vi "HEWH WT210 Data Save.vi"(10 "MW100 Data":string[][](array[string]), 11 "output cluster":T1={"Current (A):Element 1"=236.2, "Current (A):Element 2"=17.749, "Power (W):Sigma"=4192.0, "Watt Hours (Wh):Sigma"=0.0, "Voltage (V):Element 2"=236.2, "Voltage (V):Element 1"=236.2, "Current Crest Factor:Element 1"=0.0, "Current Crest Factor:Element 2"=0.0, "Voltage Harmonic (%):Element 1"=0.0, "Voltage Harmonic (%):Element 2"=0.0, "Voltage Crest Factor:Element 1"=0.0, "Voltage Crest Factor:Element 2"=0.0, "Time:Element 1"=0.0, "Frequency (Hz):Element 1"=0.0, "Apparent Power (VA):Element 1"=0.0, "Apparent Power (VA):Element 2"=0.0, "Power Factor:Element 1"=0.0, "Power Factor:Element 2"=0.0, "Max Watt Hours"=0.0, "Voltage (V):Element 2 Avg"=0.0, "Voltage (V):Element 1 Avg"=0.0} {"Voltage (V):Element 1 Avg" format="%.3g"; "Voltage (V):Element 2 Avg" format="%.3g"; "Max Watt Hours" format="%.3g"; "Power Factor:Element 2" format="%.3g"; "Power Factor:Element 1" format="%.3g"; "Apparent Power (VA):Element 2" format="%.3g"; "Apparent Power (VA):Element 1" format="%.3g"; "Frequency (Hz):Element 1" format="%.3g"; "Time:Element 1" format="%.3g"; "Voltage Crest Factor:Element 2" format="%.3g"; "Voltage Crest Factor:Element 1" format="%.3g"; "Voltage Harmonic (%):Element 2" format="%.3g"; "Voltage Harmonic (%):Element 1" format="%.3g"; "Current Crest Factor:Element 2" format="%.3g"; "Current Crest Factor:Element 1" format="%.3g"; "Voltage (V):Element 1" format="%.3g"; "Voltage (V):Element 2" format="%.3g"; "Watt Hours (Wh):Sigma" format="%.3f"; "Power (W):Sigma" format="%.3g"; "Current (A):Element 2" format="%.3e"; "Current (A):Element 1" format="%.3e"}) -> (3 "MW100 Data":string[][](array[string]))   [LabVIEW 2019]
uses:
  Utility/Type Definitions/UTILITY Power Data.ctl
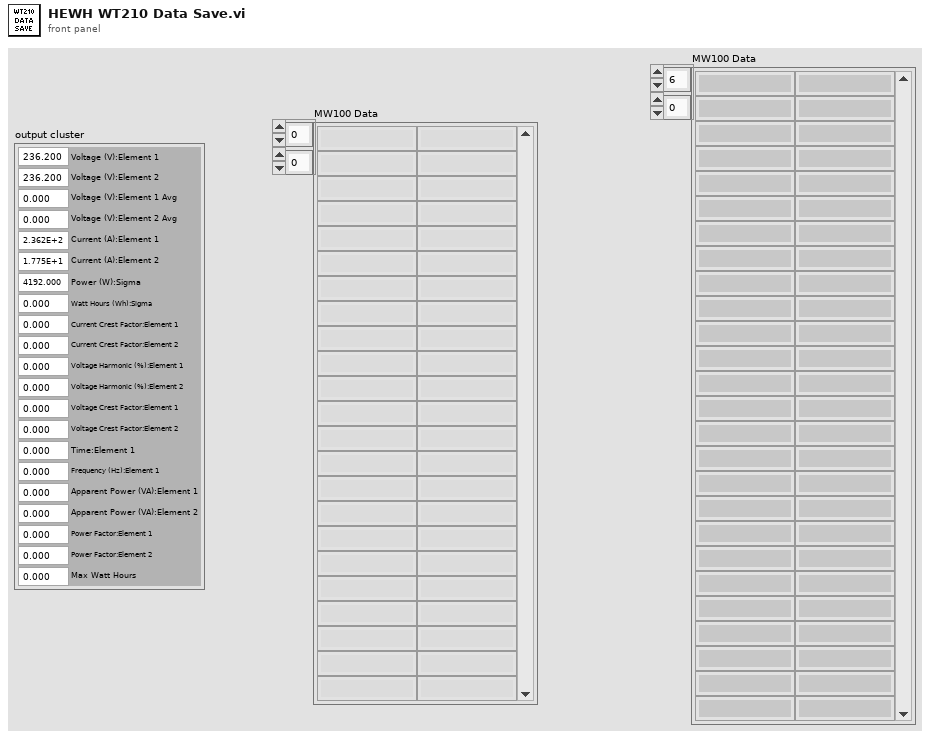
[diagram p1: front panel]
types:
  T1 = typedef "UTILITY Power Data.ctl" = cluster{"Current (A):Element 1":dbl, "Current (A):Element 2":dbl, "Power (W):Sigma":dbl, "Watt Hours (Wh):Sigma":dbl, "Voltage (V):Element 2":dbl, "Voltage (V):Element 1":dbl, "Current Crest Factor:Element 1":dbl, "Current Crest Factor:Element 2":dbl, "Voltage Harmonic (%):Element 1":dbl, "Voltage Harmonic (%):Element 2":dbl, "Voltage Crest Factor:Element 1":dbl, "Voltage Crest Factor:Element 2":dbl, "Time:Element 1":dbl, "Frequency (Hz):Element 1":dbl, "Apparent Power (VA):Element 1":dbl, "Apparent Power (VA):Element 2":dbl, "Power Factor:Element 1":dbl, "Power Factor:Element 2":dbl, "Max Watt Hours":dbl, "Voltage (V):Element 2 Avg":dbl, "Voltage (V):Element 1 Avg":dbl}
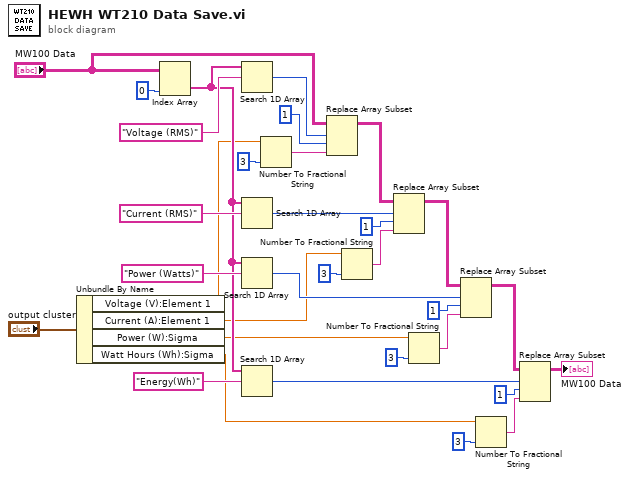
[diagram p0: block diagram]
diagram:
  n1 = Unbundle By Name("output cluster") -> ("Voltage (V):Element 1"=w16:dbl, "Current (A):Element 1"=w15:dbl, "Power (W):Sigma"=w14:dbl, "Watt Hours (Wh):Sigma"=w13:dbl)
  n2 = Index Array(array="MW100 Data", index (col)=0 ("disabled index (col)")) -> (element=w27:string[])  [unwired: 1 in]
  n3 = Search 1D Array(1D array=w27, element="Voltage (RMS)") -> (index of element=w25:i32)  [unwired: 1 in]
  n4 = Search 1D Array(1D array=w27, element="Current (RMS)") -> (index of element=w23:i32)  [unwired: 1 in]
  n5 = Search 1D Array(1D array=w27, element="Power (Watts)") -> (index of element=w20:i32)  [unwired: 1 in]
  n6 = Search 1D Array(1D array=w27, element="Energy(Wh)") -> (index of element=w19:i32)  [unwired: 1 in]
  n7 = Number To Fractional String(number=w16, precision (6)=i16 3) -> (F-format string=w8:string)  [unwired: 2 in]
  n8 = Replace Array Subset(array="MW100 Data", new element=w8, index (row)=w25, index (col)=1 ("disabled index (col)")) -> (w4:string[][])
  n9 = Number To Fractional String(number=w15, precision (6)=i16 3) -> (F-format string=w7:string)  [unwired: 2 in]
  n10 = Replace Array Subset(array=w4, new element=w7, index (row)=w23, index (col)=1 ("disabled index (col)")) -> (w3:string[][])
  n11 = Number To Fractional String(number=w14, precision (6)=i16 3) -> (F-format string=w6:string)  [unwired: 2 in]
  n12 = Replace Array Subset(array=w3, new element=w6, index (row)=w20, index (col)=1 ("disabled index (col)")) -> (w2:string[][])
  n13 = Number To Fractional String(number=w13, precision (6)=i16 3) -> (F-format string=w5:string)  [unwired: 2 in]
  n14 = Replace Array Subset(array=w2, new element=w5, index (row)=w19, index (col)=1 ("disabled index (col)")) -> (→"MW100 Data":string[][])
